vi "Init.vi"(8 "error in (no error)":errorcluster, 10 "Camera":T1, 11 "Cmd Q":refnum<queue>) -> (0 "error out":errorcluster)   [LabVIEW 2020, in "FormulaG.lvlib" / "Select Cam Cmd.lvclass"]
uses:
  Select Cam Cmd.lvclass
  FormulaG-Common/Camera.ctl
  Command/Command.lvclass
  C:/dev/SummerOfLabVIEW/sol-formulag/ProjectTemplates/Source/SummerOfLabVIEW/FormulaG/template/FormulaG/Command/Command.lvclass
  Select Cam Cmd.lvclass/Select Cam Cmd.ctl
  FormulaG-Common/FormulaG-Common.lvlib
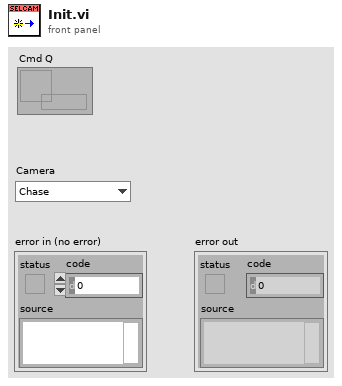
[diagram p1: front panel]
types:
  T1 = typedef "FormulaG-Common.lvlib/Camera.ctl" = enum16{"Chase", "Overhead"}
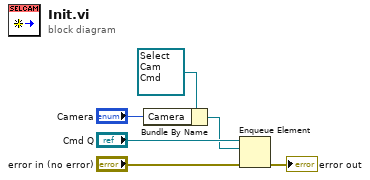
[diagram p0: block diagram]
diagram:
  n1 = Bundle By Name(cluster=refnum<class "Select Cam Cmd.lvclass"> refnum ("Select Cam Cmd in"), "Camera"="Camera") -> (w1:refnum<class "Select Cam Cmd.lvclass">)
  n2 = Enqueue Element(queue="Cmd Q", element=w1, error in (no error)="error in (no error)") -> (error out=→"error out":errorcluster)  [unwired: 1 in, 2 out]
